vi "Queue Comms Get Elements.vi"(8 "error in (no error)":errorcluster) -> (0 "error out":errorcluster, 3 "elements":T1[](array[typedef]))   [LabVIEW 2018, in "Error Handler.lvlib"]
doc: "This subVI enqueues an element in to the communications queue to be handled"
uses:
  Error Handler.lvlib
  Private Controls/Module Data.ctl
  Private Controls/Module Action.ctl
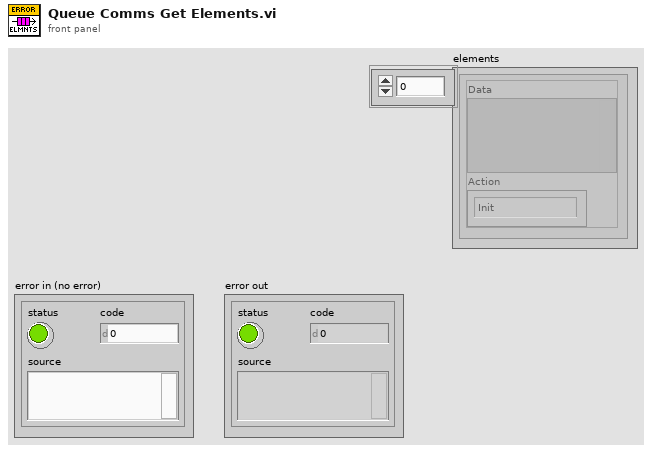
[diagram p1: front panel]
types:
  T1 = typedef "Error Handler.lvlib/Module Data.ctl" = cluster{"Data":variant, "Action":T2}
  T2 = typedef "Error Handler.lvlib/Module Action.ctl" = enum8{"Init", "Exit", "Controller Error", "UI1 Error", "UI2 Error", "UI3 Error", "File IO Error", "cRIO Error", "Calibration Error"}
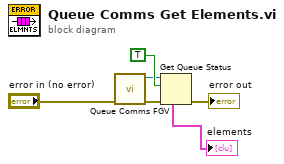
[diagram p0: block diagram]
diagram:
  n1 = call "Queue Comms FGV.vi"("error in (no error)"="error in (no error)") -> ("error out"=w3:errorcluster, "Queue out"=w4:refnum<queue>)  [unwired: 9 in]
  n2 = Get Queue Status(queue=w4, return elements? (F)=TRUE, error in (no error)=w3) -> (error out=→"error out":errorcluster, elements=→"elements":T1[])  [unwired: 6 out]
